vi "digital_number_yufan_dong.vi"(3 "Numeric Control":i32) -> (1 "Digital":T1)   [LabVIEW 2021]
uses:
  Controls/digital_number_display_yufan_dong.ctl
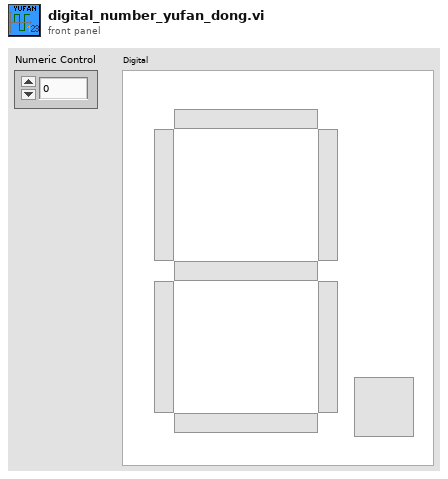
[diagram p1: front panel]
types:
  T1 = typedef "digital_number_display_yufan_dong.ctl" = cluster{"A":bool, "B":bool, "C":bool, "D":bool, "E":bool, "F":bool, "G":bool, "DP":bool}
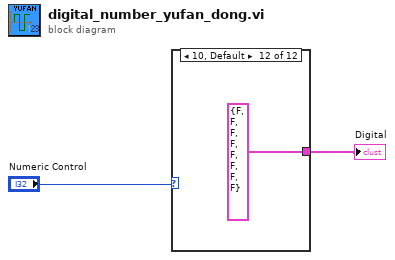
[diagram p0: block diagram]
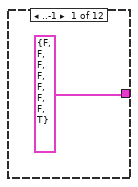
[diagram p2: hidden frame]
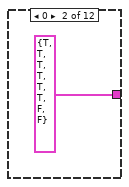
[diagram p3: hidden frame]
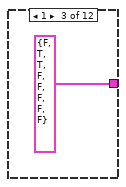
[diagram p4: hidden frame]
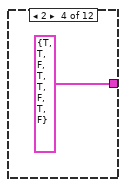
[diagram p5: hidden frame]
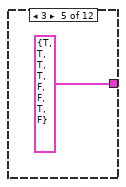
[diagram p6: hidden frame]
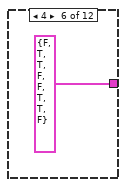
[diagram p7: hidden frame]
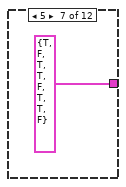
[diagram p8: hidden frame]
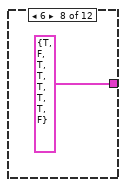
[diagram p9: hidden frame]
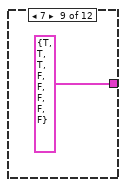
[diagram p10: hidden frame]
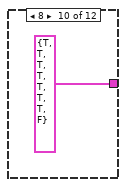
[diagram p11: hidden frame]
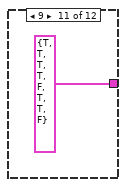
[diagram p12: hidden frame]
diagram:
  n1 = case shown="10, Default" "Numeric Control" {
    tunnel: [T1 {"A"=FALSE, "B"=FALSE, "C"=FALSE, "D"=FALSE, "E"=FALSE, "F"=FALSE, "G"=FALSE, "DP"=TRUE} ("Cluster 2") T1 {"A"=TRUE, "B"=TRUE, "C"=TRUE, "D"=TRUE, "E"=TRUE, "F"=TRUE, "G"=FALSE, "DP"=FALSE} ("Cluster 2") T1 {"A"=FALSE, "B"=TRUE, "C"=TRUE, "D"=FALSE, "E"=FALSE, "F"=FALSE, "G"=FALSE, "DP"=FALSE} ("Cluster 2") T1 {"A"=TRUE, "B"=TRUE, "C"=FALSE, "D"=TRUE, "E"=TRUE, "F"=FALSE, "G"=TRUE, "DP"=FALSE} ("Cluster 2") T1 {"A"=TRUE, "B"=TRUE, "C"=TRUE, "D"=TRUE, "E"=FALSE, "F"=FALSE, "G"=TRUE, "DP"=FALSE} ("Cluster 2") T1 {"A"=FALSE, "B"=TRUE, "C"=TRUE, "D"=FALSE, "E"=FALSE, "F"=TRUE, "G"=TRUE, "DP"=FALSE} ("Cluster 2") T1 {"A"=TRUE, "B"=FALSE, "C"=TRUE, "D"=TRUE, "E"=FALSE, "F"=TRUE, "G"=TRUE, "DP"=FALSE} ("Cluster 2") T1 {"A"=TRUE, "B"=FALSE, "C"=TRUE, "D"=TRUE, "E"=TRUE, "F"=TRUE, "G"=TRUE, "DP"=FALSE} ("Cluster 2") T1 {"A"=TRUE, "B"=TRUE, "C"=TRUE, "D"=FALSE, "E"=FALSE, "F"=FALSE, "G"=FALSE, "DP"=FALSE} ("Cluster 2") T1 {"A"=TRUE, "B"=TRUE, "C"=TRUE, "D"=TRUE, "E"=TRUE, "F"=TRUE, "G"=TRUE, "DP"=FALSE} ("Cluster 2") T1 {"A"=TRUE, "B"=TRUE, "C"=TRUE, "D"=TRUE, "E"=FALSE, "F"=TRUE, "G"=TRUE, "DP"=FALSE} ("Cluster 2") T1 {"A"=FALSE, "B"=FALSE, "C"=FALSE, "D"=FALSE, "E"=FALSE, "F"=FALSE, "G"=FALSE, "DP"=FALSE} ("Cluster 2")] -> w1
    frame ..-1 {
    }
    frame 0 {
    }
    frame 1 {
    }
    frame 2 {
    }
    frame 3 {
    }
    frame 4 {
    }
    frame 5 {
    }
    frame 6 {
    }
    frame 7 {
    }
    frame 8 {
    }
    frame 9 {
    }
    frame 10, Default {
    }
  }
  "Digital" <- w1
